vi "超标留样自动校时.vi"   [LabVIEW 2016, in "超标留样集成.lvlib" / "ESTD1200.lvlib"]
uses:
  ESTD1200.lvlib
  <vilib>/Plasmionique/MB Master/MB Master.lvlib
types:
  T1 = cluster{"采样器状态":u16, "采样模式":u16, "瓶数":u16, "采样量":u16, "当前瓶号":u16, "当前进程":u16, "采样瓶状态":cluster{"1号瓶":bool, "2号瓶":bool, "3号瓶":bool, "4号瓶":bool, "5号瓶":bool, "6号瓶":bool, "7号瓶":bool, "8号瓶":bool, "9号瓶":bool, "10号瓶":bool, "11号瓶":bool, "12号瓶":bool}, "门锁状态":bool, "冰箱当前温度":sgl, "系统时间":timestamp}
  T2 = typedef "LVDateTimeRec.ctl" = cluster{"秒数的小数部分":dbl, "秒":i32, "分":i32, "时":i32, "日":i32, "月":i32, "年":i32, "天数（周）":i32, "天数（年）":i32, "DST":i32}
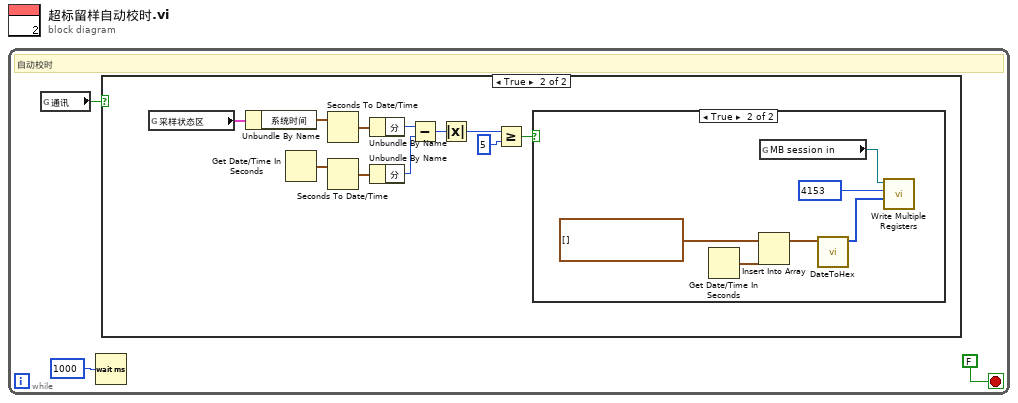
[diagram p0: block diagram]
diagram:
  n1 = while {
    stop <- FALSE stop-if-true
    # "自动校时"
    n2 = global read "超标留样全局.vi" "通讯"() -> (w1:bool)
    n3 = Wait (ms)(milliseconds to wait=u32 1000 ("等待时间（毫秒）")) -> ()  [unwired: 1 out]
    n4 = case shown="True" w1 {
      frame False {
      }
      frame True {
        n5 = global read "超标留样全局.vi" "采样状态区"() -> (w14:T1)
        n6 = Unbundle By Name(w14) -> ("系统时间"=w13:timestamp)
        n7 = Get Date/Time In Seconds() -> (seconds since 1Jan1904=w11:timestamp)
        n8 = Seconds To Date/Time(time stamp (now)=w13) -> (date time rec=w12:T2)  [unwired: 1 in]
        n9 = Seconds To Date/Time(time stamp (now)=w11) -> (date time rec=w10:T2)  [unwired: 1 in]
        n10 = Unbundle By Name(w12) -> ("分"=w9:i32)
        n11 = Unbundle By Name(w10) -> ("分"=w8:i32)
        n12 = Subtract(x=w9, y=w8) -> (x-y=w6:i32)
        n13 = Absolute Value(x=w6) -> (abs(x)=w5:i32)
        n14 = Greater Or Equal?(x=w5, y=5) -> (x >= y?=w4:bool)
        n15 = case shown="True" w4 {
          frame False {
          }
          frame True {
            n16 = Get Date/Time In Seconds() -> (seconds since 1Jan1904=w16:timestamp)
            n17 = Insert Into Array(array=timestamp[] [] ("数组"), new element=w16) -> (w18:timestamp[])  [unwired: 1 in]
            n18 = global read "超标留样全局.vi" "MB session in"() -> (w20:refnum<class "MB_Master.lvclass">)
            n19 = call "DateToHex.vi"("数组输入"=w18) -> ("数组输出"=w15:u16[])  [unwired: 10 in]
            n20 = call <vilib>:"Write Multiple Registers.vi"("values"=w15, "starting address"=u16 4153, "MB session in"=w20) -> ()  [unwired: 7 in, 2 out]
          }
        }
      }
    }
  }
